vi "MccHat_Main.vi"() -> ()   [LabVIEW 2019]
uses:
  MccHat_Global.vi
panel:
  in  "n_sample":i16=20 caption="Sample"
  in  "clear_chart":bool=TRUE caption="Clear charts to start"
  out "P":dbl caption="Magnet Pressure" format="%.2f"
  out "Last Meas. Time":timestamp format="%<%Y-%m-%d %H:%M:%S>T"
  in  "Tab Control":enum32{"Pressure", "Raw Voltage"}(tab)
  out "chart_pres":waveform(dbl)[](graph)=[{"t0"=timestamp(3772890114.31303 s since 1904-01-01), "dt"=1.0, "Y"=[0.8687935985565186]}, {"t0"=timestamp(3772890114.31303 s since 1904-01-01), "dt"=1.0, "Y"=[86.87935985565186]}, {"t0"=timestamp(3772890114.31303 s since 1904-01-01), "dt"=1.0, "Y"=[30.48853325313992]}, {"t0"=timestamp(3772890114.31303 s since 1904-01-01), "dt"=1.0, "Y"=[303.6385332531399]}]
  out "chart_raw_v":waveform(dbl)[](graph)=[{"t0"=timestamp(3785686355.130285 s since 1904-01-01), "dt"=1.0, "Y"=[-0.00251999]}, {"t0"=timestamp(3785686355.130285 s since 1904-01-01), "dt"=1.0, "Y"=[-0.00346989]}]
  out "name":string caption="Name"
  in  "interval":u32=2000 caption="Interval"
  out "status_init":bool caption="Initialization"
  out "status_read":bool caption="Readout"
  in  "stop":bool
  in  "port":u16=1111 caption="Port"
  in  "address":string="192.168.24.203" caption="IP Addr."
  # "MCC HAT #01"
  # "ms"
  # "per read"
  # "psig"
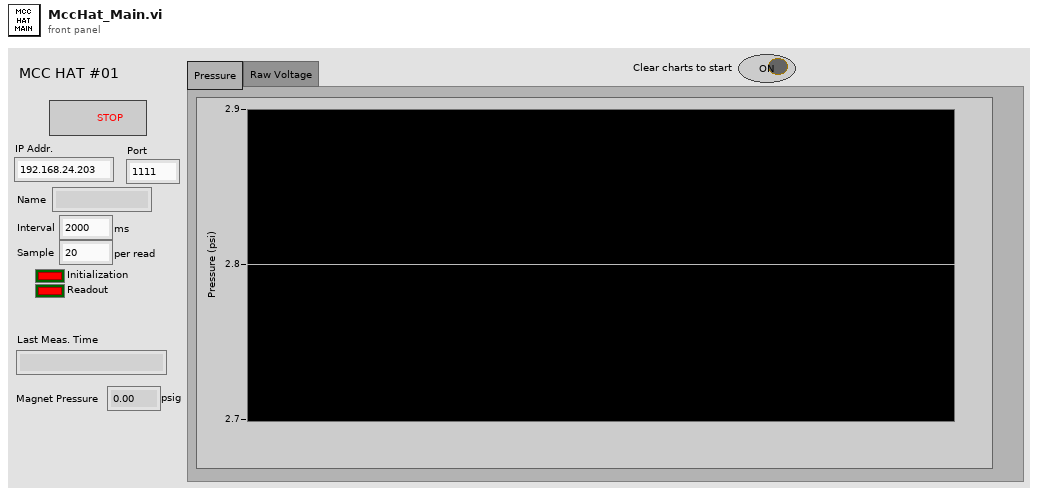
[diagram p1: front panel]
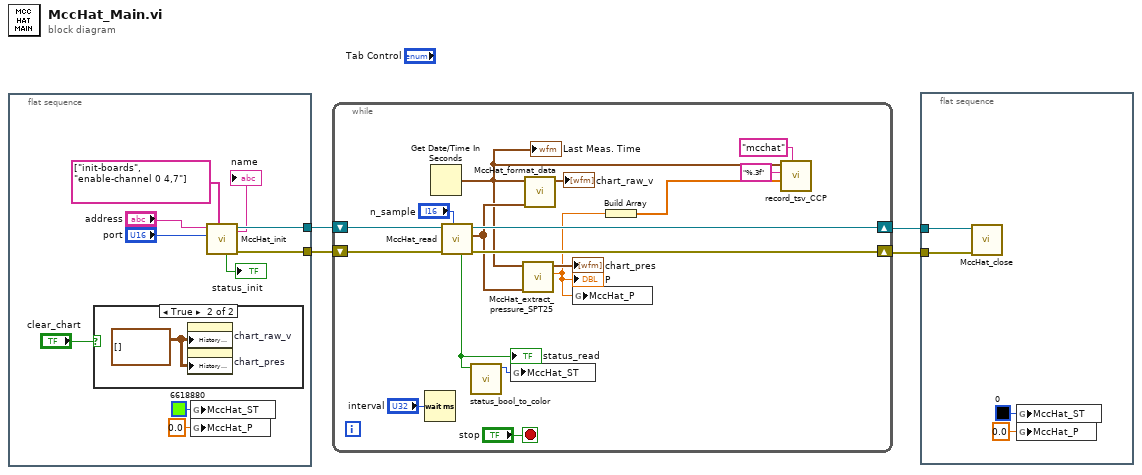
[diagram p0: block diagram]
diagram:
  n1 = flat-sequence {
    tunnel: [w12] -> w4
    tunnel: [w11] -> w3
    frame #0 {
      n2 = case shown="True" "clear_chart" {
        frame False {
        }
        frame True {
          w15 = waveform(dbl)[][] [] ("History Data")
          n3 = property on="chart_raw_v" class="WFChart (strict)"("History Data"=w15) -> ()  [unwired: 2 in, 2 out]
          n4 = property on="chart_pres" class="WFChart (strict)"("History Data"=w15) -> ()  [unwired: 2 in, 2 out]
        }
      }
      n5 = global write "MccHat_Global.vi" "MccHat_ST"(u32 6618880 ("LJT4_ST")) -> ()
      n6 = global write "MccHat_Global.vi" "MccHat_P"(0.0 ("MccHat_P")) -> ()
      n7 = call "MccHat_init.vi"("commands"=string[] ["init-boards", "enable-channel 0 4,7"], "port"="port", "address"="address") -> ("error out"=w11:errorcluster, "conn_id"=w12:refnum<k5>, "status"=→"status_init":bool, "server"=→"name":string)  [unwired: 5 in]
    }
  }
  n8 = while {
    shift-right: [w28] -> w1
    shift-left: w4 -> [w30]
    shift-right: [w27] -> w2
    shift-left: w3 -> [w29]
    stop <- "stop" stop-if-true
    n9 = Wait (ms)(milliseconds to wait="interval") -> ()  [unwired: 1 out]
    n10 = Get Date/Time In Seconds() -> (seconds since 1Jan1904=w21:timestamp)
    "Last Meas. Time" <- w21
    n11 = call "MccHat_read.vi"("n_read"="n_sample", "error in"=w29, "conn_id_in"=w30) -> ("error out"=w27:errorcluster, "readings"=w26:cluster{i32, i32, dbl}[], "conn_id_out"=w28:refnum<k5>, "status"=w22:bool)  [unwired: 5 in]
    "status_read" <- w22
    n12 = call "status_bool_to_color.vi"("status_bool_1"=w22) -> ("status_color"=w23:u32)  [unwired: 10 in]
    n13 = global write "MccHat_Global.vi" "MccHat_ST"(w23) -> ()
    n14 = call "MccHat_extract_pressure_SPT25.vi"("readings"=w26, "time"=w21) -> ("P"=w20:dbl, "waveform_array"=→"chart_pres":waveform(dbl)[])  [unwired: 8 in]
    "P" <- w20
    n15 = call "MccHat_format_data.vi"("readings"=w26, "time"=w21) -> ("waveform_array_A"=→"chart_raw_v":waveform(dbl)[])  [unwired: 9 in]
    n16 = global write "MccHat_Global.vi" "MccHat_P"(w20) -> ()
    n17 = Build Array(w20) -> (w19:dbl[])
    n18 = call "record_tsv_CCP.vi"("folder_name"="mcchat", "value_array"=w19, "format"="%.3f", "time"=w21) -> ()  [unwired: 6 in, 2 out]
  }
  n19 = flat-sequence {
    tunnel: w2 -> [w36]
    tunnel: w1 -> [w35]
    frame #0 {
      n20 = call "MccHat_close.vi"("error in"=w36, "conn_id"=w35) -> ()  [unwired: 8 in, 2 out]
      n21 = global write "MccHat_Global.vi" "MccHat_ST"(u32 0 ("LJT4_ST")) -> ()
      n22 = global write "MccHat_Global.vi" "MccHat_P"(0.0 ("MccHat_P")) -> ()
    }
  }
